vi "ADQ214 Get Record Size.vi"(8 "error in (no error)":errorcluster, 10 "adq214_num":i32, 11 "adq_cu_ptr":u32) -> (0 "error out":errorcluster, 2 "function return":u32, 3 "adq_cu_ptr out":u32)   [LabVIEW 2013, in "ADQAPI.lvlib"]
doc: "extern \"C\" __declspec(dllimport) unsigned int ADQ214_GetRecordSize(void* adq_cu_ptr, int adq214_num);"
uses:
  LabView_ADQ214_summer2015/ADQAPI.lvlib
  ADQAPI.dll
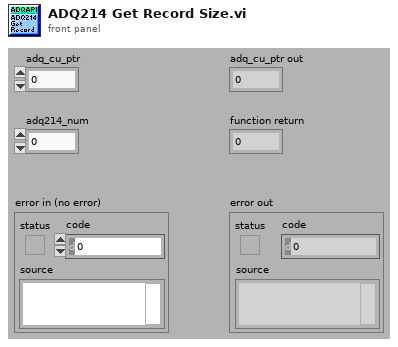
[diagram p1: front panel]
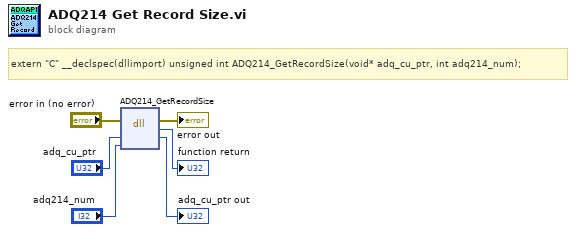
[diagram p0: block diagram]
diagram:
  # "extern \"C\" __declspec(dllimport) unsigned int\tADQ214_GetRecordSize(void* adq_cu_ptr, int adq214_num);"
  n1 = dll-call lib="C:/Users/astafiev/Desktop/Ilya/LabView_Radion/ADQAPI.*" fn="ADQ214_GetRecordSize"(error in="error in (no error)", "adq_cu_ptr"="adq_cu_ptr", "adq214_num"="adq214_num") -> (error out=→"error out":errorcluster, →"function return":u32, "adq_cu_ptr"=→"adq_cu_ptr out":u32)  [unwired: 3 in, 1 out]
